vi "Do_Every_minute.vi"(1 "Ch Names":string[](array[string]), 2 "Values":dbl[](array[numeric]) format="%.2f") -> ()   [LabVIEW 2013]
uses:
  Do_Every_5mins.ctl
  Anemometry/Anemometry Sub Vis/Controls/In_Range.ctl
  ADAM Client/Sub VIs/ADAM Controls/Traverse_Level_State.ctl
  ADAM Client/Sub VIs/ADAM Controls/Valco_valve_ph.ctl
  ADAM_Global.vi
panel:
  in  "Disable Sending email to estates regarding Chilled water Temp":bool=TRUE
  in  "Max K Factor":dbl=2.7
  out "Case":T1
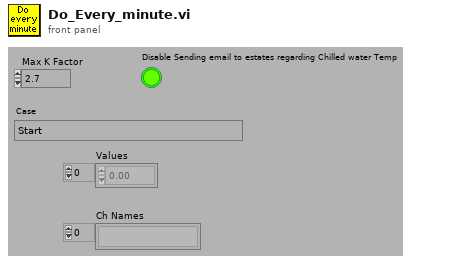
[diagram p1: front panel]
types:
  T1 = typedef "Do_Every_5mins.ctl" = enum16{"Start", "Update EnFlo Tunnel Speed Tweak", "Are EnFlo Tun Fan Bearings too Hot?", "Check EnFlo tweak factor?", "Are Inlet Screens Blocked?", "Tweak demanded chilled water temp", "Is Dew point meter Alive?", "Condensation Occurring", "Condensation Alert", "More checks", "Set FFID Valve to Measure", "End"}
  T2 = typedef "In_Range.ctl" = enum16{"%", "±", "% & ±"}
  T3 = typedef "Traverse_Level_State.ctl" = enum16{"Running", "Complete"}
  T4 = typedef "Client_State_Cluster.ctl" = cluster{"Client Name":string, "Traverse level State":T3, "People to Email":string[], "Next Contact Time":dbl}
  T5 = typedef "Valco_valve_ph.ctl" = u16
  T6 = cluster{"second":i32, "minute":i32, "hour":i32, "day of month":i32, "month":i32, "year":i32, "day of week":i32, "day of year":i32, "is DST":i32}
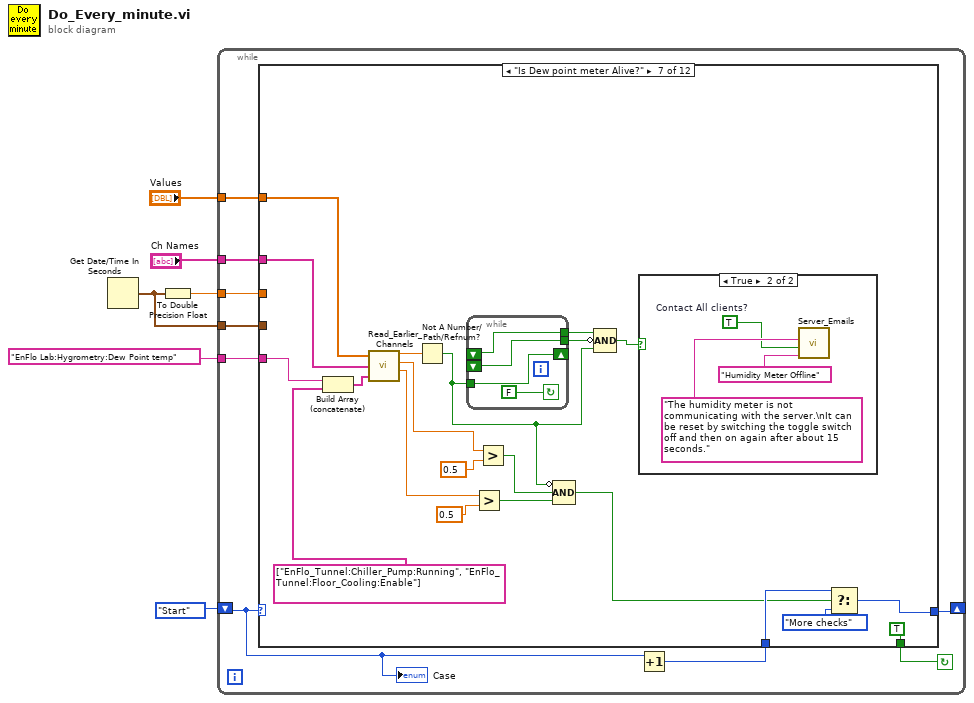
[diagram p0: block diagram]
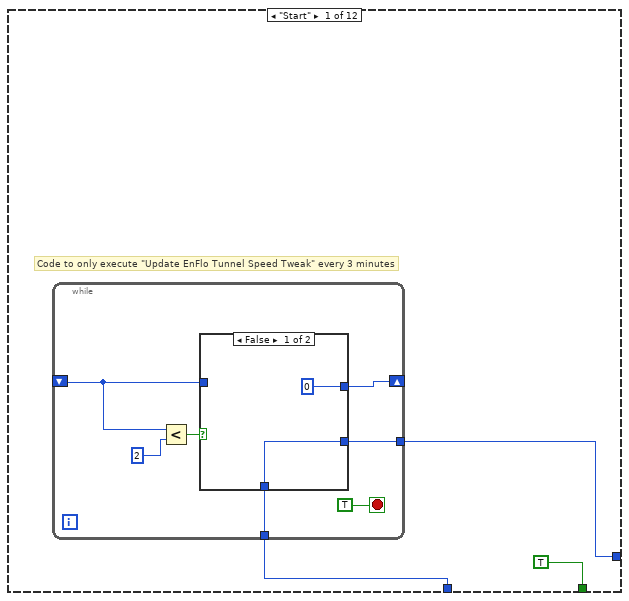
[diagram p2: hidden frame]
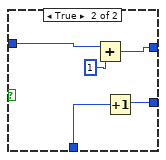
[diagram p3: hidden frame]
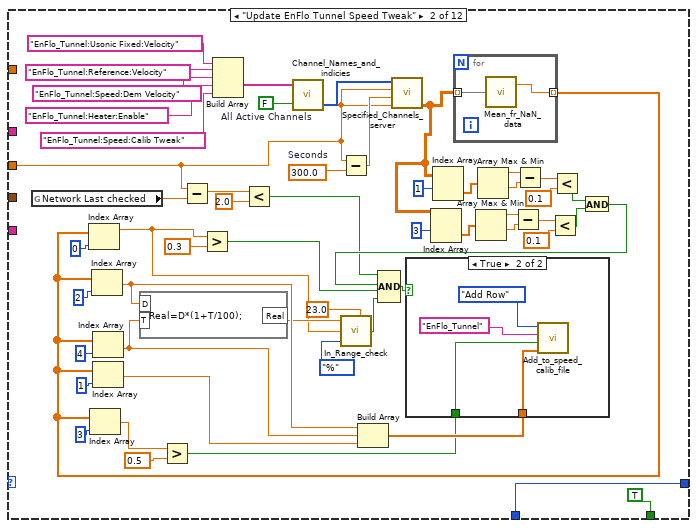
[diagram p4: hidden frame]
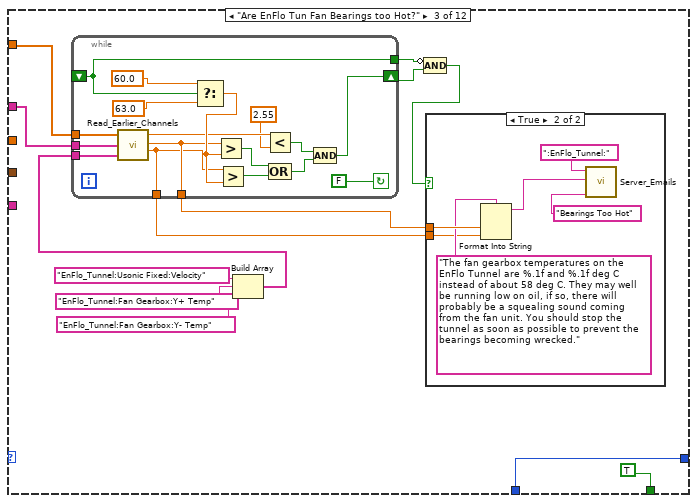
[diagram p6: hidden frame]
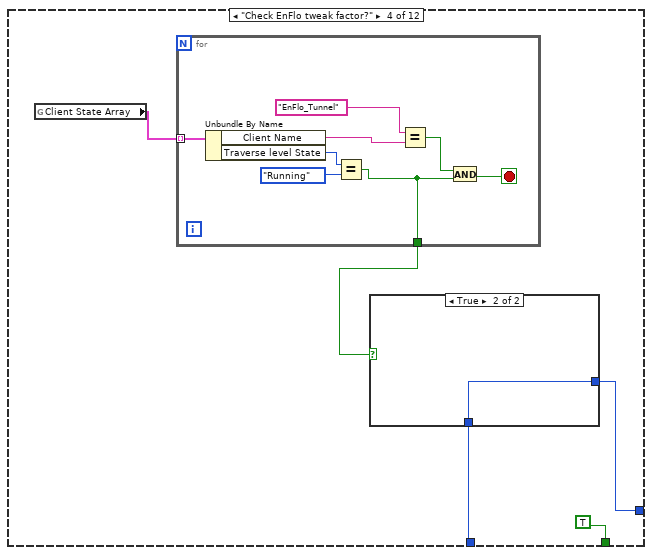
[diagram p8: hidden frame]
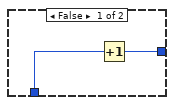
[diagram p9: hidden frame]
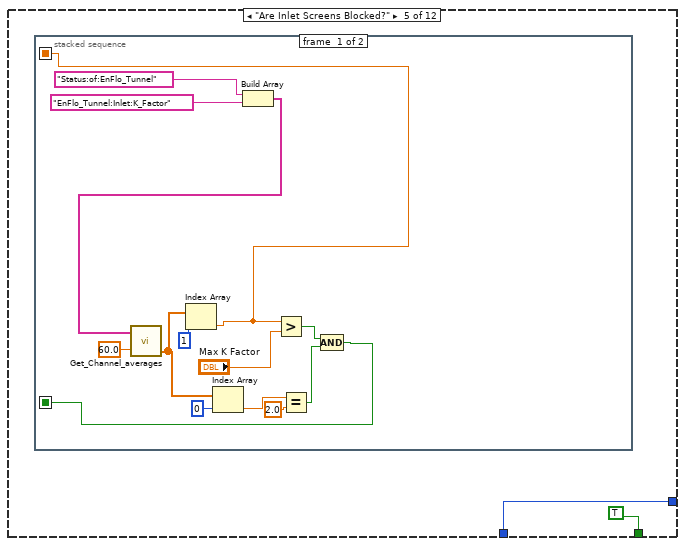
[diagram p10: hidden frame]
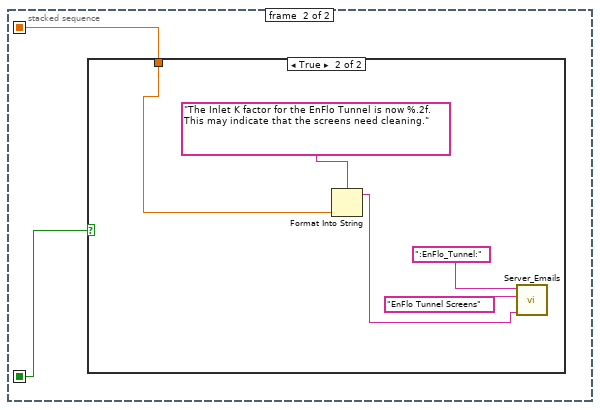
[diagram p11: hidden frame]
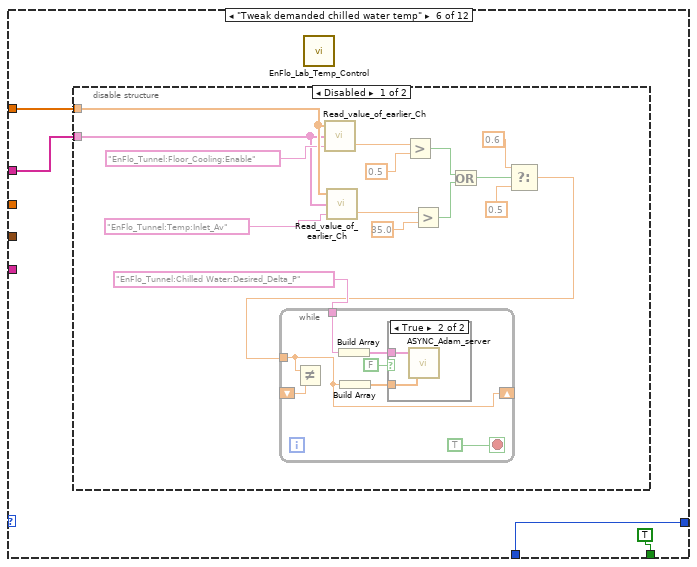
[diagram p13: hidden frame]
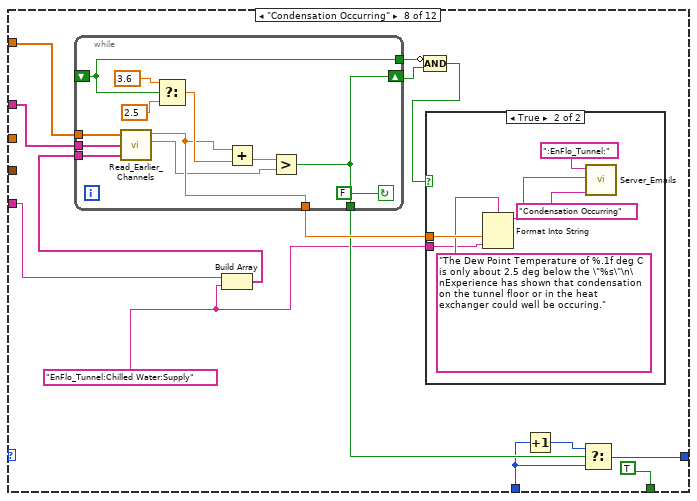
[diagram p17: hidden frame]
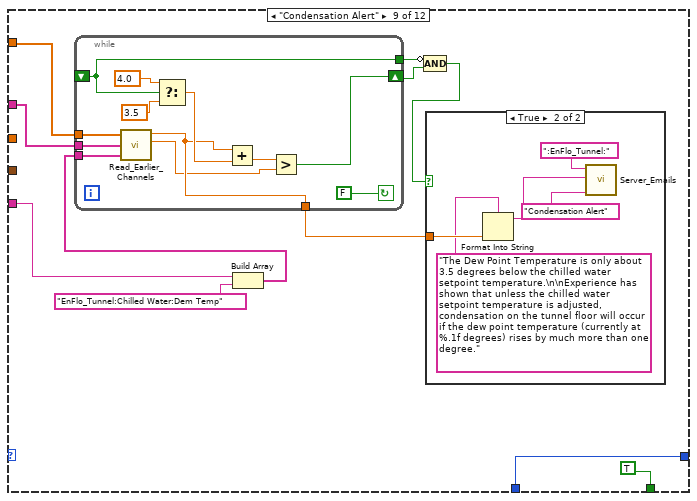
[diagram p19: hidden frame]
diagram:
  n1 = Get Date/Time In Seconds() -> (seconds since 1Jan1904=w1:timestamp)
  n2 = To Double Precision Float(number=w1) -> (double precision float=w2:dbl)
  n3 = while {
    tunnel: "EnFlo Lab:Hygrometry:Dew Point temp" -> [w9]
    tunnel: "Values" -> [w13]
    tunnel: "Ch Names" -> [w14]
    shift-left: Do_Every_5mins."Start" ("Case") -> [w10]
    shift-right: [w11] -> _
    tunnel: w2 -> [w8]
    tunnel: w1 -> [w7]
    stop <- w15 continue-if-true
    n4 = Increment(x=w10) -> (x+1=w12:T1)
    n5 = case shown="\"Is Dew point meter Alive?\"" w10 {
      tunnel: [TRUE TRUE TRUE TRUE TRUE TRUE TRUE TRUE TRUE TRUE TRUE FALSE] -> w15
      tunnel: w14 -> [_ _ w102 _ _ w168 w212 w235 w262 w305 w312 w345]
      tunnel: w13 -> [_ _ w103 _ _ w169 w213 w236 w263 w306 w311 w344]
      tunnel: w12 -> [w16 w74 w93 w131 w145 w171 w206 w226 w265 w303 w330 w348]
      tunnel: [w17 w74 w93 w130 w145 w171 w216 w227 w265 w302 w330 w348] -> w11
      tunnel: w9 -> [_ _ _ _ _ _ w211 w229 w256 _ _ _]
      tunnel: w8 -> [_ w34 _ _ _ _ _ _ _ _ w329 _]
      tunnel: w7 -> [_ _ _ _ _ _ _ _ _ _ _ w346]
      frame "Start" {
        # "Code to only execute \"Update EnFlo Tunnel Speed Tweak\" every 3 minutes"
        n6 = while {
          shift-right: [w22] -> _
          shift-left: _ -> [w19]
          tunnel: [w21] -> w17
          tunnel: w16 -> [w20]
          stop <- TRUE stop-if-true
          n7 = Less?(x=w19, y=2) -> (x < y?=w23:bool)
          n8 = case shown="False" w23 {
            tunnel: [0 w30] -> w22
            tunnel: [w26 w28] -> w21
            tunnel: w20 -> [w26 w29]
            tunnel: w19 -> [_ w31]
            frame False {
            }
            frame True {
              n9 = Add(x=w31, y=1) -> (x+y=w30:i32)
              n10 = Increment(x=w29) -> (x+1=w28:T1)
            }
          }
        }
      }
      frame "Update EnFlo Tunnel Speed Tweak" {
        w68 = 300.0  # Seconds
        w70 = FALSE  # All Active Channels
        n11 = global read "ADAM_Global.vi" "Network Last checked"() -> (w35:dbl)
        n12 = Subtract(x=w34, y=w35) -> (x-y=w36:dbl)
        n13 = Build Array("EnFlo_Tunnel:Usonic Fixed:Velocity", "EnFlo_Tunnel:Reference:Velocity", "EnFlo_Tunnel:Speed:Dem Velocity", "EnFlo_Tunnel:Heater:Enable", "EnFlo_Tunnel:Speed:Calib Tweak") -> (w67:string[])
        n14 = Less?(x=w36, y=2.0) -> (x < y?=w33:bool)
        n15 = call "Channel_Names_and_indicies.vi"("All Active Channels"=w70, "Desired Ch Names"=w67) -> ("Indicies"=w69:i32[])  [unwired: 1 out]
        n16 = Subtract(x=w34, y=w68) -> (x-y=w66:dbl)
        n17 = call "Specified_Channels_server.vi"("End time"=w34, "Start time"=w66, "Clients time"=w34, "Requested channels"=w69) -> ("Output array"=w48:dbl[][])  [unwired: 1 in, 4 out]
        n18 = Index Array(array=w48, index (row)=3 ("Index")) -> (element=w50:dbl[])  [unwired: 1 in]
        n19 = Index Array(array=w48, index (row)=1 ("Index")) -> (element=w64:dbl[])  [unwired: 1 in]
        n20 = for {
          tunnel: w48 -> [w88] mode=indexing
          tunnel: [w87] -> w57 mode=indexing
          n21 = call "Mean_fr_NaN_data.vi"("Data"=w88) -> ("Mean value"=w87:dbl)  [unwired: 1 out]
        }
        n22 = Index Array(array=w57, index=0) -> (element=w41:dbl)
        n23 = Index Array(array=w57, index=3) -> (element=w77:dbl)
        n24 = Index Array(array=w57, index=2) -> (element=w43:dbl)
        n25 = Index Array(array=w57, index=4) -> (element=w44:dbl)
        n26 = Index Array(array=w57, index=1) -> (element=w55:dbl)
        n27 = formula code="Real=D*(1+T/100);"("D"=w43, "T"=w44) -> ("Real"=w42:dbl)
        n28 = Greater?(x=w77, y=0.5) -> (0:w56:bool)
        n29 = Greater?(x=w41, y=0.3) -> (0:w75:bool)
        n30 = call "In_Range_check.vi"("%"=23.0, "Mode"=In_Range."%", "Value"=w41, "Setpoint"=w42) -> ("In Range"=w38:bool)  [unwired: 1 in, 2 out]
        n31 = Build Array(w43, w44, w55) -> (w72:dbl[])
        n32 = Array Max & Min(array=w50) -> (max value=w51:dbl, min value=w52:dbl)  [unwired: 2 out]
        n33 = Array Max & Min(array=w64) -> (max value=w63:dbl, min value=w62:dbl)  [unwired: 2 out]
        n34 = Subtract(x=w51, y=w52) -> (x-y=w53:dbl)
        n35 = Subtract(x=w63, y=w62) -> (x-y=w61:dbl)
        n36 = Less?(x=w53, y=0.1) -> (x < y?=w47:bool)
        n37 = Less?(x=w61, y=0.1) -> (x < y?=w46:bool)
        n38 = And(x=w46, y=w47) -> (x .and. y?=w45:bool)
        n39 = Compound Arithmetic op=AND(w33, w45, w75, w38) -> (w71:bool)
        n40 = case shown="True" w71 {
          tunnel: w72 -> [_ w91]
          tunnel: w56 -> [_ w90]
          frame False {
          }
          frame True {
            n41 = call "Add_to_speed_calib_file.vi"("New Row"=w91, "Tunnel Heated?"=w90, "Rig Name"="EnFlo_Tunnel" ("y"), "Mode"=enum16{"Add Row", "Get Error Value"}."Add Row") -> ()  [unwired: 2 in, 2 out]
          }
        }
      }
      frame "Are EnFlo Tun Fan Bearings too Hot?" {
        n42 = Build Array("EnFlo_Tunnel:Usonic Fixed:Velocity", "EnFlo_Tunnel:Fan Gearbox:Y+ Temp", "EnFlo_Tunnel:Fan Gearbox:Y- Temp") -> (w101:string[])
        n43 = while {
          tunnel: [w107] -> w94
          tunnel: [w108] -> w95
          tunnel: [w117] -> w100
          shift-left: _ -> [w117]
          shift-right: [w109] -> w99
          tunnel: w101 -> [w120]
          tunnel: w102 -> [w121]
          tunnel: w103 -> [w122]
          stop <- FALSE continue-if-true
          n44 = call "Read_Earlier_Channels.vi"("Present scan array"=w122, "Ch names"=w121, "Desired Channels"=w120) -> ("Index 0"=w115:dbl, "Index 1"=w108:dbl, "Index 2"=w107:dbl)  [unwired: 3 out]
          n45 = Select(t=60.0, s=w117, f=63.0) -> (s? t:f=w116:dbl)
          n46 = Greater?(x=w108, y=w116) -> (0:w113:bool)
          n47 = Greater?(x=w107, y=w116) -> (0:w112:bool)
          n48 = Less?(x=w115, y=2.55) -> (x < y?=w111:bool)
          n49 = Compound Arithmetic op=OR(w113, w112) -> (w110:bool)
          n50 = Compound Arithmetic op=AND(w111, w110) -> (w109:bool)
        }
        n51 = Compound Arithmetic op=AND(invert w100, w99) -> (w98:bool)
        n52 = case shown="True" w98 {
          tunnel: w95 -> [_ w126]
          tunnel: w94 -> [_ w123]
          frame False {
          }
          frame True {
            n53 = Format Into String(format string="The fan gearbox temperatures on the EnFlo Tunnel are %.1f and %.1f deg C instead of about 58 deg C. They may well be running low on oil, if so, there will probably be a squealing sound coming from the fan unit. You should stop the tunnel as soon as possible to prevent the bearings becoming wrecked." ("Format String"), w126, w123) -> (resulting string=w125:string)  [unwired: 2 in, 1 out]
            n54 = call "Server_Emails.vi"("Client Name Contains"=":EnFlo_Tunnel:", "Message"=w125, "Subject"="Bearings Too Hot" ("Error Type")) -> ()  [unwired: 2 in, 3 out]
          }
        }
      }
      frame "Check EnFlo tweak factor?" {
        n55 = global read "ADAM_Global.vi" "Client State Array"() -> (w132:T4[])
        n56 = for {
          tunnel: w132 -> [w144] mode=indexing
          tunnel: [w137] -> w129
          stop <- w138 stop-if-true
          n57 = Unbundle By Name(w144) -> ("Client Name"=w140:string, "Traverse level State"=w143:T3)
          n58 = Equal?(x=w143, y=Traverse_Level_State."Running" ("Traverse level State")) -> (x = y?=w137:bool)
          n59 = Equal?(x="EnFlo_Tunnel" ("y"), y=w140) -> (x = y?=w139:bool)
          n60 = And(x=w139, y=w137) -> (x .and. y?=w138:bool)
        }
        n61 = case shown="True" w129 {
          tunnel: w131 -> [w135 w136]
          tunnel: [w134 w136] -> w130
          frame False {
            n62 = Increment(x=w135) -> (x+1=w134:T1)
          }
          frame True {
          }
        }
      }
      frame "Are Inlet Screens Blocked?" {
        n63 = stacked-sequence {
          seq-local: [w147 _] -> [_ w162]
          seq-local: [w150 _] -> [_ w161]
          frame #0 {
            n64 = Build Array("Status:of:EnFlo_Tunnel", "EnFlo_Tunnel:Inlet:K_Factor") -> (w152:string[])
            n65 = call "Get_Channel_averages.vi"("Desired Ch Names"=w152, "Averaging time (mins)"=60.0) -> ("number"=w158:dbl[])  [unwired: 1 in, 2 out]
            n66 = Index Array(array=w158, index=1) -> (element=w147:dbl)
            n67 = Index Array(array=w158, index=0) -> (element=w157:dbl)
            n68 = Greater?(x=w147, y="Max K Factor") -> (0:w149:bool)
            n69 = Equal?(x=w157, y=2.0) -> (x = y?=w155:bool)
            n70 = Compound Arithmetic op=AND(w149, w155) -> (w150:bool)
          }
          frame #1 {
            n71 = case shown="True" w161 {
              tunnel: w162 -> [_ w166]
              frame False {
              }
              frame True {
                n72 = Format Into String(format string="The Inlet K factor for the EnFlo Tunnel is now %.2f. This may indicate that the screens need cleaning." ("Format String"), w166) -> (resulting string=w164:string)  [unwired: 2 in, 1 out]
                n73 = call "Server_Emails.vi"("Client Name Contains"=":EnFlo_Tunnel:", "Message"="EnFlo Tunnel Screens", "Subject"=w164) -> ()  [unwired: 2 in, 3 out]
              }
            }
          }
        }
      }
      frame "Tweak demanded chilled water temp" {
        n74 = disable-structure shown="Disabled" {
          disable-tunnel: w169 -> [w185 _]
          disable-tunnel: w168 -> [w183 _]
          frame Disabled {
            n75 = call "Read_value_of_earlier_Ch.vi"("Desired Ch to Read"="EnFlo_Tunnel:Floor_Cooling:Enable", "Ch names"=w183, "Present scan array"=w185) -> ("Value"=w181:dbl)  [unwired: 1 in, 1 out]
            n76 = call "Read_value_of_earlier_Ch.vi"("Desired Ch to Read"="EnFlo_Tunnel:Temp:Inlet_Av", "Ch names"=w183, "Present scan array"=w185) -> ("Value"=w179:dbl)  [unwired: 1 in, 1 out]
            n77 = Greater?(x=w181, y=0.5) -> (0:w177:bool)
            n78 = Greater?(x=w179, y=35.0) -> (0:w176:bool)
            n79 = Or(x=w177, y=w176) -> (x .or. y?=w175:bool)
            n80 = Select(t=0.6, s=w175, f=0.5 ("t")) -> (s? t:f=w172:dbl)
            n81 = while {
              shift-right: [w189] -> _
              shift-left: _ -> [w190]
              tunnel: w172 -> [w189]
              tunnel: "EnFlo_Tunnel:Chilled Water:Desired_Delta_P" -> [w191]
              stop <- TRUE stop-if-true
              n82 = Not Equal?(x=w189, y=w190) -> ()  [unwired: 1 out]
              n83 = Build Array(w191) -> (w192:string[])
              n84 = Build Array(w189) -> (w193:dbl[])
              n85 = case shown="True" FALSE {
                tunnel: w193 -> [_ w195]
                tunnel: w192 -> [_ w194]
                frame False {
                }
                frame True {
                  n86 = call "ASYNC_Adam_server.vi"("Values"=w195, "Channel Names"=w194) -> ()  [unwired: 1 in, 3 out]
                }
              }
            }
          }
          frame Enabled {
          }
        }
        n87 = call "EnFlo_Lab_Temp_Control.vi"() -> ()  [unwired: 1 out]
      }
      frame "Is Dew point meter Alive?" {
        n88 = Build Array (concatenate)(w211, string[] ["EnFlo_Tunnel:Chiller_Pump:Running", "EnFlo_Tunnel:Floor_Cooling:Enable"] ("appended array")) -> (w210:string[])
        n89 = call "Read_Earlier_Channels.vi"("Present scan array"=w213, "Ch names"=w212, "Desired Channels"=w210) -> ("Index 0"=w209:dbl, "Index 1"=w208:dbl, "Index 2"=w197:dbl)  [unwired: 3 out]
        n90 = Not A Number/Path/Refnum?(number/path/refnum=w209) -> (NaN/Path/Refnum?=w203:bool)
        n91 = while {
          tunnel: [w218] -> w201
          tunnel: [w219] -> w202
          shift-left: _ -> [w219]
          tunnel: w203 -> [w220]
          shift-left: _ -> [w218]
          shift-right: [w220] -> _
          stop <- FALSE continue-if-true
        }
        n92 = Greater?(x=w197, y=0.5) -> (0:w196:bool)
        n93 = Greater?(x=w208, y=0.5) -> (0:w207:bool)
        n94 = Compound Arithmetic op=AND(invert w203, w207, w196) -> (w204:bool)
        n95 = Compound Arithmetic op=AND(w201, invert w202, w203) -> (w214:bool)
        n96 = case shown="True" w214 {
          frame False {
          }
          frame True {
            w221 = TRUE  # Contact All clients?
            n97 = call "Server_Emails.vi"("Message"="The humidity meter is not communicating with the server.\nIt can be reset by switching the toggle switch off and then on again after about 15 seconds." ("Bundle Element"), "Contact All clients?"=w221, "Subject"="Humidity Meter Offline" ("Error Type")) -> ()  [unwired: 2 in, 3 out]
          }
        }
        n98 = Select(t=w206, s=w204, f=Do_Every_5mins."More checks" ("Case")) -> (s? t:f=w216:T1)
      }
      frame "Condensation Occurring" {
        w224 = "EnFlo_Tunnel:Chilled Water:Supply"
        n99 = Build Array(w229, w224) -> (w234:string[])
        n100 = while {
          tunnel: [w239] -> w228
          tunnel: [w241] -> w230
          tunnel: [w242] -> w233
          shift-left: _ -> [w242]
          shift-right: [w239] -> w232
          tunnel: w234 -> [w247]
          tunnel: w235 -> [w248]
          tunnel: w236 -> [w249]
          stop <- FALSE continue-if-true
          n101 = call "Read_Earlier_Channels.vi"("Present scan array"=w249, "Ch names"=w248, "Desired Channels"=w247) -> ("Index 0"=w241:dbl, "Index 1"=w240:dbl)  [unwired: 4 out]
          n102 = Select(t=3.6, s=w242, f=2.5) -> (s? t:f=w243:dbl)
          n103 = Add(x=w241, y=w243) -> (x+y=w246:dbl)
          n104 = Greater?(x=w246, y=w240) -> (0:w239:bool)
        }
        n105 = Compound Arithmetic op=AND(invert w233, w232) -> (w231:bool)
        n106 = case shown="True" w231 {
          tunnel: w230 -> [_ w253]
          tunnel: w224 -> [_ w250]
          frame False {
          }
          frame True {
            n107 = Format Into String(format string="The Dew Point Temperature of %.1f deg C is only about 2.5 deg below the \"%s\"\n\nExperience has shown that condensation on the tunnel floor or in the heat exchanger could well be occuring." ("Format String"), w253, w250) -> (resulting string=w252:string)  [unwired: 2 in, 1 out]
            n108 = call "Server_Emails.vi"("Client Name Contains"=":EnFlo_Tunnel:", "Message"=w252, "Subject"="Condensation Occurring" ("Error Type")) -> ()  [unwired: 2 in, 3 out]
          }
        }
        n109 = Increment(x=w226) -> (x+1=w225:T1)
        n110 = Select(t=w225, s=w228, f=w226) -> (s? t:f=w227:T1)
      }
      frame "Condensation Alert" {
        n111 = Build Array(w256, "EnFlo_Tunnel:Chilled Water:Dem Temp") -> (w261:string[])
        n112 = while {
          tunnel: [w269] -> w257
          tunnel: [w271] -> w260
          shift-left: _ -> [w271]
          shift-right: [w270] -> w259
          tunnel: w261 -> [w276]
          tunnel: w262 -> [w277]
          tunnel: w263 -> [w278]
          stop <- FALSE continue-if-true
          n113 = call "Read_Earlier_Channels.vi"("Present scan array"=w278, "Ch names"=w277, "Desired Channels"=w276) -> ("Index 0"=w269:dbl, "Index 1"=w268:dbl)  [unwired: 4 out]
          n114 = Select(t=4.0, s=w271, f=3.5) -> (s? t:f=w272:dbl)
          n115 = Add(x=w269, y=w272) -> (x+y=w275:dbl)
          n116 = Greater?(x=w275, y=w268) -> (0:w270:bool)
        }
        n117 = Compound Arithmetic op=AND(invert w260, w259) -> (w258:bool)
        n118 = case shown="True" w258 {
          tunnel: w257 -> [_ w281]
          frame False {
          }
          frame True {
            n119 = Format Into String(format string="The Dew Point Temperature is only about 3.5 degrees below the chilled water setpoint temperature.\n\nExperience has shown that unless the chilled water setpoint temperature is adjusted, condensation on the tunnel floor will occur if the dew point temperature (currently at %.1f degrees) rises by much more than one degree." ("Format String"), w281) -> (resulting string=w280:string)  [unwired: 2 in, 1 out]
            n120 = call "Server_Emails.vi"("Client Name Contains"=":EnFlo_Tunnel:", "Message"=w280, "Subject"="Condensation Alert" ("Error Type")) -> ()  [unwired: 2 in, 3 out]
          }
        }
      }
      frame "More checks" {
        w285 = "EnFlo_Tunnel:Extra_Lights:Enable"
        n121 = Build Array("Fast FID:Valco Valve:Position", "Status:of:EnFlo_Tunnel", w285) -> (w300:string[])
        n122 = call "Read_Earlier_Channels.vi"("Present scan array"=w306, "Ch names"=w305, "Desired Channels"=w300) -> ("Index 0"=w293:dbl, "Index 1"=w291:dbl, "Index 2"=w289:dbl)  [unwired: 3 out]
        n123 = Greater?(x=w289, y=0.5) -> (0:w287:bool)
        n124 = Equal?(x=w291, y=2.0) -> (x = y?=w286:bool)
        n125 = And(x=w286, y=w287) -> (x .and. y?=w284:bool)
        n126 = case shown="True" w284 {
          tunnel: w285 -> [_ w310]
          frame False {
          }
          frame True {
            n127 = Build Array(w310) -> (w309:string[])
            n128 = call "ASYNC_Adam_server.vi"("Values"=dbl[] [0.0], "Channel Names"=w309) -> ()  [unwired: 1 in, 3 out]
          }
        }
        n129 = Equal?(x=4.0, y=w293) -> (x = y?=w297:bool)
        n130 = Equal?(x=1.0, y=w293) -> (x = y?=w296:bool)
        n131 = Not A Number/Path/Refnum?(number/path/refnum=w293) -> (NaN/Path/Refnum?=w298:bool)
        n132 = Compound Arithmetic op=OR(w296, w297, w298) -> (w295:bool)
        n133 = Select(t=Do_Every_5mins."End" ("Case"), s=w295, f=w303) -> (s? t:f=w302:T1)
      }
      frame "Set FFID Valve to Measure" {
        w328 = FALSE  # All Active Channels
        n134 = Build Array("Fast FID:Valco Valve:Position") -> (w326:string[])
        n135 = call "Channel_Names_and_indicies.vi"("All Active Channels"=w328, "Desired Ch Names"=w326) -> ("Indicies"=w327:i32[])  [unwired: 1 out]
        n136 = Subtract(x=w329, y=700.0) -> (x-y=w324:dbl)
        n137 = call "Specified_Channels_server.vi"("End time"=w329, "Start time"=w324, "Clients time"=w329, "Requested channels"=w327) -> ("Output array"=w321:dbl[][])  [unwired: 1 in, 4 out]
        n138 = Index Array(array=w321, index (row)=0 ("Index")) -> (element=w317:dbl[])  [unwired: 1 in]
        n139 = Not A Number/Path/Refnum?(number/path/refnum=w317) -> (NaN/Path/Refnum?=w316:bool[])
        n140 = Or Array Elements(Boolean array=w316) -> (logical OR=w314:bool)
        n141 = Array Max & Min(array=w317) -> (max value=w319:dbl, min value=w320:dbl)  [unwired: 2 out]
        n142 = Subtract(x=w319, y=w320) -> (x-y=w318:dbl)
        n143 = Equal To 0?(x=w318) -> (x = 0?=w315:bool)
        n144 = Compound Arithmetic op=AND(w315, invert w314) -> (w313:bool)
        n145 = case shown="True" w313 {
          tunnel: w312 -> [_ w338]
          tunnel: w311 -> [_ w337]
          frame False {
          }
          frame True {
            n146 = Build Array("FFID:System:Enable") -> (w335:string[])
            n147 = call "Read_Earlier_Channels.vi"("Present scan array"=w337, "Ch names"=w338, "Desired Channels"=w335) -> ("Index 0"=w334:dbl)  [unwired: 5 out]
            n148 = Greater?(x=w334, y=0.5) -> (0:w332:bool)
            n149 = case shown="True" w332 {
              frame False {
                n150 = Build Array(0.0) -> (w340:dbl[])
                n151 = Build Array("GMU:Gas:Enable") -> (w342:string[])
                n152 = call "ASYNC_Adam_client.vi"("Values"=w340, "Channel Names"=w342) -> ()  [unwired: 2 out]
              }
              frame True {
                w343 = T5 4 items=["", "Zero Air", "Calib 1", "Calib 2", "Measure"] ("Requested Position")
                n153 = call "Fast_FID_Valve_Control.vi"("Requested Position"=w343) -> ()  [unwired: 7 out]
              }
            }
          }
        }
      }
      frame "End" {
        n154 = stacked-sequence {
          seq-local: [w355 _] -> [_ w375]
          seq-local: [w349 _] -> [_ w372]
          tunnel: w346 -> [w360 _]
          tunnel: w345 -> [w352 w374]
          tunnel: w344 -> [w353 w373]
          frame #0 {
            n155 = call <vilib>:"LV70TimeStampToDateRec.vi"("time stamp"=w360) -> ("date time rec"=w361:T6)
            n156 = Unbundle By Name(w361) -> ("hour"=w359:i32, "day of week"=w358:i32)
            n157 = while {
              tunnel: w359 -> [w371]
              tunnel: w358 -> [w369]
              shift-right: [w364] -> w356
              shift-left: _ -> [w363]
              tunnel: [w363] -> w357
              stop <- FALSE continue-if-true
              n158 = Equal?(x=w371, y=10) -> (x = y?=w365:bool)
              n159 = In Range and Coerce(upper limit=7, x=w369, lower limit=1) -> (In Range?=w366:bool)  [unwired: 1 out]
              n160 = And(x=w365, y=w366) -> (x .and. y?=w364:bool)
            }
            n161 = call "Read_value_of_earlier_Ch.vi"("Desired Ch to Read"="Uni:Chilled Water:Temp", "Ch names"=w352, "Present scan array"=w353) -> ("Value"=w349:dbl)  [unwired: 1 in, 1 out]
            n162 = Greater?(x=w349, y=15.0) -> (0:w350:bool)
            n163 = Compound Arithmetic op=AND(w350, invert w357, w356) -> (w355:bool)
          }
          frame #1 {
            n164 = case shown="True" w375 {
              tunnel: w374 -> [_ _]
              tunnel: w373 -> [_ _]
              tunnel: w372 -> [_ w383]
              frame False {
              }
              frame True {
                n165 = Select(t=string[] [], s="Disable Sending email to estates regarding Chilled water Temp", f=string[] ["efmenquiries@surrey.ac.uk"] ("Extra People to Email")) -> (s? t:f=w376:string[])
                n166 = Format Into String(format string="Dear Estates\n\nThe monitoring system in the EnFlo Lab (01AB01) is currently indicating that the Chilled water in the AB Building is at %d deg C.\n\nPlease could you arrange for somebody to come and investigate this please.\n\nThanks very much\n\nPaul Hayden x9545  or Mobile  07961 608409", w383) -> (resulting string=w382:string)  [unwired: 2 in, 1 out]
                n167 = call "Server_Emails.vi"("Message"=w382, "Contact All clients?"=TRUE, "Subject"="Chilled water in AB Building above 15 deg C" ("Error Type"), "Extra People to Email"=w376) -> ()  [unwired: 1 in, 3 out]
              }
            }
          }
        }
      }
    }
    "Case" <- w10
  }
